vi "Retry TCP.vi"(7 "error in (no error)":errorcluster, 8 "Numeric":i32, 11 "String":string) -> (6 "error out":errorcluster)   [LabVIEW 2020]
uses:
  Global variable.vi
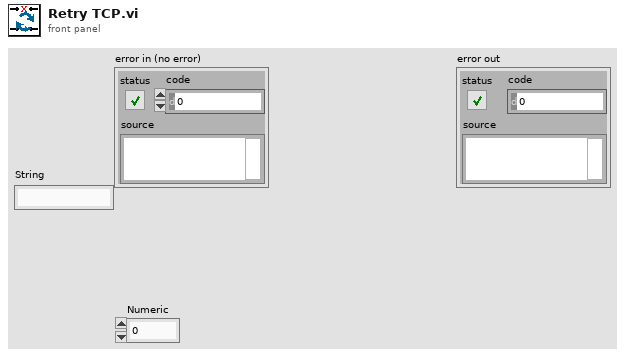
[diagram p1: front panel]
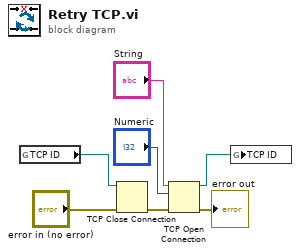
[diagram p0: block diagram]
diagram:
  n1 = global read "Global variable.vi" "TCP ID"() -> (w7:refnum<k5>)
  n2 = TCP Close Connection(connection ID=w7, error in (no error)="error in (no error)") -> (error out=w6:errorcluster)  [unwired: 1 in, 1 out]
  n3 = TCP Open Connection(address="String", remote port or service name="Numeric", error in (no error)=w6) -> (connection ID=w3:refnum<k5>, error out=→"error out":errorcluster)  [unwired: 2 in]
  n4 = global write "Global variable.vi" "TCP ID"(w3) -> ()
